vi "locate function.vi"(8 "error in":errorcluster, 10 "index":i32, 11 "tag bus processing plugin module configuration in":refnum<class "tag bus processing plugin module configuration.lvclass">) -> (0 "error out":errorcluster, 1 "found":bool, 2 "processing function":T1, 3 "tag bus processing plugin module configuration out":refnum<class "tag bus processing plugin module configuration.lvclass">)   [LabVIEW 2013, in "tag bus processing plugin editor node.lvclass"]
uses:
  tag bus processing plugin editor node.lvclass
  module/configuration/tag bus processing plugin module configuration.lvclass
  module/configuration/processing channels.ctl
  <vilib>/NI/Tag Bus Module Framework/channel/TBM channel.lvclass
  module/configuration/tag bus processing plugin module configuration.lvclass/tag bus processing plugin module configuration.ctl
  module/configuration/Read functions.vi
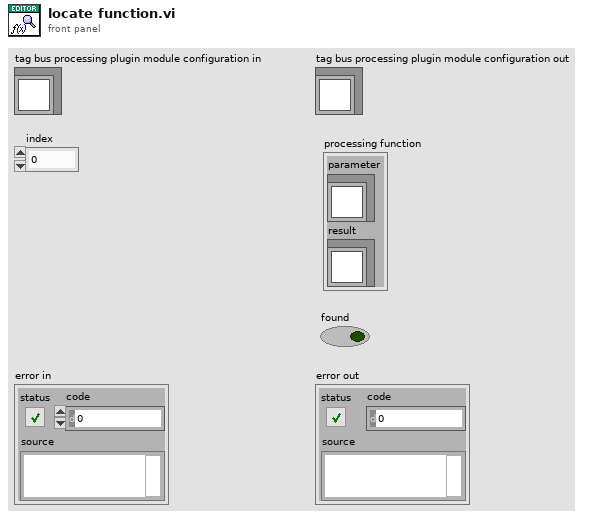
[diagram p1: front panel]
types:
  T1 = typedef "tag bus processing plugin module configuration.lvclass/processing channels.ctl" = cluster{"parameter":refnum<class "TBM channel.lvclass">, "result":refnum<class "TBM channel.lvclass">}
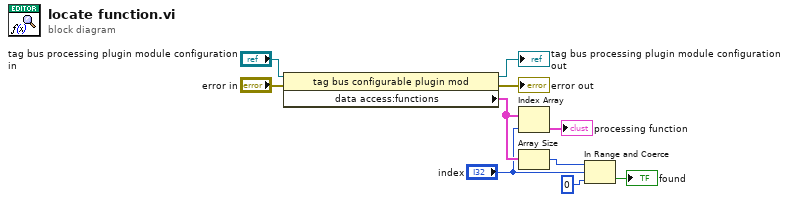
[diagram p0: block diagram]
diagram:
  n1 = property class="tag bus configurable plugin mod"(reference="tag bus processing plugin module configuration in", error in="error in") -> (reference out=→"tag bus processing plugin module configuration out":refnum<class "tag bus processing plugin module configuration.lvclass">, error out=→"error out":errorcluster, "data access:functions"=w3:T1[])
  n2 = Index Array(array=w3, index="index") -> (element=→"processing function":T1)
  n3 = Array Size(array=w3) -> (size(s)=w6:i32)
  n4 = In Range and Coerce(upper limit=w6, x="index", lower limit=0) -> (In Range?=→"found":bool)  [unwired: 1 out]
